vi "图像排孔校正.vi"() -> ()   [LabVIEW 2018]
uses:
  <vilib>/vision/Calibration.llb/Distortion Model.ctl
  <vilib>/vision/Calibration.llb/Distortion Model Types.ctl
  <vilib>/vision/NI_Vision_Development_Module.lvlib
panel:
  out "error out":errorcluster
  out "Image 2":T1(plugin-control)
  out "Image":T1(plugin-control)
  in  "路径":path
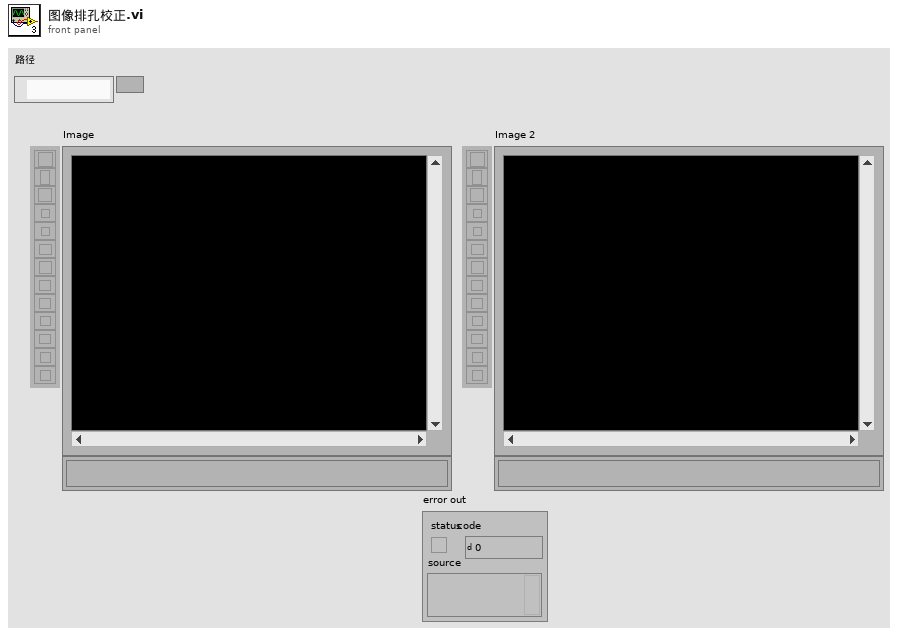
[diagram p1: front panel]
types:
  T1 = typedef "IMAQ Image.ctl" = refnum<image>
  T2 = cluster{"Corrected Image Scaling":u32, "Corrected Image Learn ROI":u32, "Learn Correction Table?":bool}
  T3 = typedef "Distortion Model.ctl" = cluster{"Distortion Model":T4, "Polynomial Model Setup":cluster{"Radial Coefficient":u32, "Tangential Coefficients ":bool}}
  T4 = typedef "Distortion Model Types.ctl" = i32
  T5 = typedef "Image Unit" = enum32{"Undefined", "Angström", "Micrometer", "Millimeter", "Centimeter", "Meter", "Kilometer", "Microinch", "Inch", "Feet", "Nautical miles", "Standard miles", "Steps"}
  T6 = typedef "Calibration Reference Points.ctl" = cluster{"Pixel Coordinates":cluster{"X":dbl, "Y":dbl}[], "Real World Coordinates":cluster{"X":dbl, "Y":dbl}[], "Unit":T5, "Image Size":cluster{"X":u32, "Y":u32}}
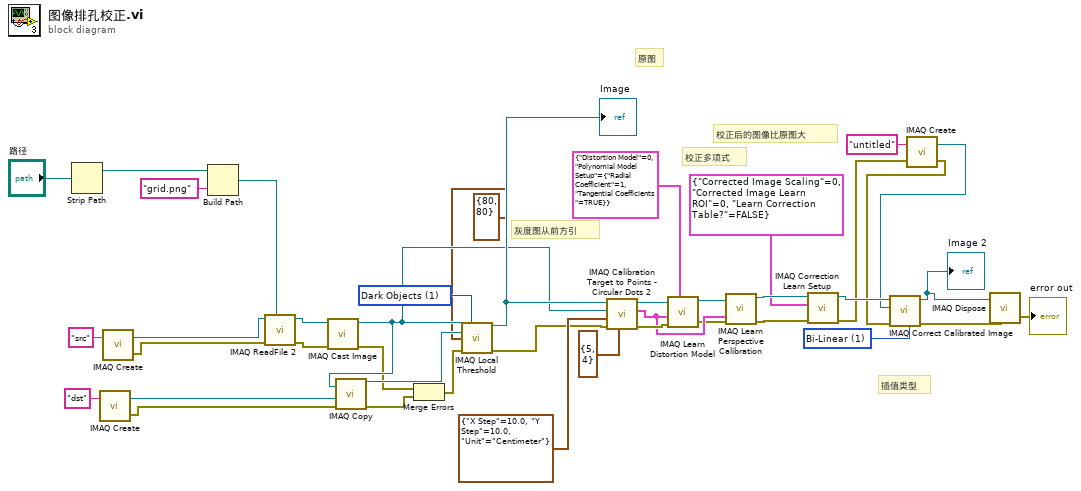
[diagram p0: block diagram]
diagram:
  w12 = u32 1 items=["Zero Order", "Bi-Linear", "Quadratic", "Cubic Spline"] ("Interpolation Type")
  w28 = u32 1 items=["Bright Objects", "Dark Objects"] ("Look For (Bright Objects)")
  # "校正后的图像比原图大"
  # "插值类型"
  # "原图"
  # "校正多项式"
  # "灰度图从前方引"
  n1 = Strip Path(path="路径") -> (stripped path=w40:path)  [unwired: 1 out]
  n2 = call "IMAQ Create"("Image Name"="dst") -> ("New Image"=w7:T1, "error out"=w31:errorcluster)  [unwired: 4 in]
  n3 = call "IMAQ Create"("Image Name"="src") -> ("New Image"=w37:T1, "error out"=w35:errorcluster)  [unwired: 4 in]
  n4 = Build Path(base path=w40, name or relative path="grid.png" ("名称或相对路径")) -> (appended path=w38:path)
  n5 = call "IMAQ ReadFile 2"("File Path"=w38, "error in (no error)"=w35, "Image"=w37) -> ("error out"=w33:errorcluster, "Image Out"=w34:T1)  [unwired: 4 in, 3 out]
  n6 = call "IMAQ Cast Image"("error in (no error)"=w33, "Image Src"=w34) -> ("error out"=w4:errorcluster, "Image Dst Out"=w6:T1)  [unwired: 8 in]
  n7 = call "IMAQ Copy"("error in (no error)"=w31, "Image Dst"=w7, "Image Src"=w6) -> ("error out"=w29:errorcluster, "Image Dst Out"=w30:T1)  [unwired: 3 in]
  n8 = Merge Errors(w4, w29) -> (w3:errorcluster)
  n9 = call "IMAQ Local Threshold"("Image Src"=w6, "Look For (Bright Objects)"=w28, "Image Dst"=w30, "Window Size (32x32)"=cluster{"SizeX":i32, "SizeY":i32} {"SizeX"=80, "SizeY"=80}, "error in (no error)"=w3) -> ("Image Dst Out"=w8:T1, "error out"=w2:errorcluster)  [unwired: 9 in]
  "Image" <- w8
  n10 = call "IMAQ Calibration Target to Points - Circular Dots 2"("Grid Size"=cluster{"Max X":u32, "Max Y":u32} {"Max X"=5, "Max Y"=4}, "error in (no error)"=w2, "Grid Descriptor"=cluster{"X Step":sgl, "Y Step":sgl, "Unit":T5} {"X Step"=10.0, "Y Step"=10.0, "Unit"=enum."Centimeter"}, "Grayscale Image"=w6, "Target Image"=w8) -> ("error out"=w24:errorcluster, "Reference Points"=w22:T6, "Target Image (dup)"=w25:T1)  [unwired: 4 in]
  n11 = call "IMAQ Learn Distortion Model"("Distortion Model Setup"=T3 {"Distortion Model"=0, "Polynomial Model Setup"={"Radial Coefficient"=1, "Tangential Coefficients "=TRUE}}, "error in (no error)"=w24, "Reference Points"=w22, "Calibration Template Image"=w25) -> ("error out"=w21:errorcluster, "Calibration Template Image Out"=w5:T1)  [unwired: 6 in]
  n12 = call "IMAQ Learn Perspective Calibration"("error in (no error)"=w21, "Reference Points"=w22, "Calibration Template Image"=w5) -> ("error out"=w20:errorcluster, "Calibration Template Image Out"=w19:T1)  [unwired: 7 in]
  n13 = call "IMAQ Correction Learn Setup"("error in (no error)"=w20, "Correction Learn Setup"=T2 {"Corrected Image Scaling"=0, "Corrected Image Learn ROI"=0, "Learn Correction Table?"=FALSE}, "Calibration Template Image"=w19) -> ("error out"=w15:errorcluster, "Calibration Template Image Out"=w17:T1)  [unwired: 7 in]
  n14 = call "IMAQ Create"("Image Name"="untitled", "error in (no error)"=w15) -> ("New Image"=w13:T1, "error out"=w14:errorcluster)  [unwired: 3 in]
  n15 = call "IMAQ Correct Calibrated Image"("Interpolation Type"=w12, "error in (no error)"=w14, "Image Dst"=w13, "Image Src"=w17) -> ("error out"=w10:errorcluster, "Corrected Image"=w11:T1)  [unwired: 6 in]
  "Image 2" <- w11
  n16 = call "IMAQ Dispose"("Image"=w11, "error in (no error)"=w10) -> ("error out"=→"error out":errorcluster)  [unwired: 4 in]
